vi "RichToFlatcif_plugincore_TimingStatistics.vi"(5 "OutputClusterType":T1, 11 "InputCluster":T3) -> (3 "OutputCluster":T1)   [LabVIEW 2021, in "CIF_Manager_client.lvlib"]
uses:
  CIF_Manager_client.lvlib
  cif_plugincore_TimingStatistics.ctl
  cif_plugincore_TimingStatsBasic.ctl
  cif_plugincore_TimingStatistics_Flat.ctl
  cif_plugincore_TimingStatsBasic_Flat.ctl
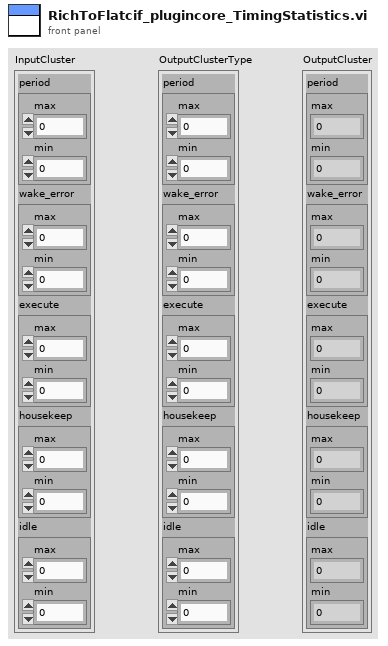
[diagram p1: front panel]
types:
  T1 = typedef "CIF_Manager_client.lvlib/cif_plugincore_TimingStatistics_Flat.ctl" = cluster{"period":T2, "wake_error":T2, "execute":T2, "housekeep":T2, "idle":T2}
  T2 = typedef "CIF_Manager_client.lvlib/cif_plugincore_TimingStatsBasic_Flat.ctl" = cluster{"max":i32, "min":i32}
  T3 = typedef "CIF_Manager_client.lvlib/cif_plugincore_TimingStatistics.ctl" = cluster{"period":T4, "wake_error":T4, "execute":T4, "housekeep":T4, "idle":T4}
  T4 = typedef "CIF_Manager_client.lvlib/cif_plugincore_TimingStatsBasic.ctl" = cluster{"max":i32, "min":i32}
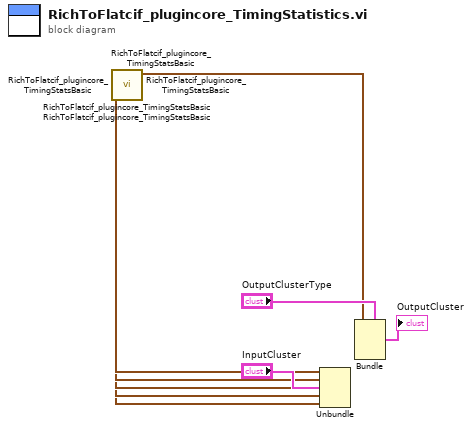
[diagram p0: block diagram]
diagram:
  n1 = Unbundle "Unbundle"("InputCluster") -> ("period"=w10:T4, "wake_error"=w8:T4, "execute"=w6:T4, "housekeep"=w4:T4, "idle"=w2:T4)
  n2 = call "RichToFlatcif_plugincore_TimingStatsBasic.vi"("InputCluster"=w2) -> ("OutputCluster"=w1:T2)  [unwired: 10 in]
  n3 = call "RichToFlatcif_plugincore_TimingStatsBasic.vi"("InputCluster"=w4) -> ("OutputCluster"=w3:T2)  [unwired: 10 in]
  n4 = call "RichToFlatcif_plugincore_TimingStatsBasic.vi"("InputCluster"=w6) -> ("OutputCluster"=w5:T2)  [unwired: 10 in]
  n5 = call "RichToFlatcif_plugincore_TimingStatsBasic.vi"("InputCluster"=w8) -> ("OutputCluster"=w7:T2)  [unwired: 10 in]
  n6 = call "RichToFlatcif_plugincore_TimingStatsBasic.vi"("InputCluster"=w10) -> ("OutputCluster"=w9:T2)  [unwired: 10 in]
  n7 = Bundle "Bundle"(cluster="OutputClusterType", "period"=w9, "wake_error"=w7, "execute"=w5, "housekeep"=w3, "idle"=w1) -> (→"OutputCluster":T1)
